vi "Set Remote Sensors.vi"(10 "Robot Sensors In":T1[](array[typedef]) {"Kobuki Sensors"."Infrared" format="%02x"; "iRobot Sensors"."Infrared" format="%02x"; "accelerometer"."z axis (g)" format="%.3f"; "accelerometer"."y axis (g)" format="%.3f"; "accelerometer"."x axis (g)" format="%.3f"}, 11 "Communication Refs":T14[](array[typedef])) -> ()   [LabVIEW 2014]
uses:
  iRobot Remote Ref.ctl
  iRobot/Sensor/Sensor Group 6.ctl
  iRobot/Sensor/Bumps + Wheel Drops.ctl
  iRobot/Sensor/Buttons.ctl
  iRobot/Sensor/Charging State.ctl
  iRobot/Sensor/Charging Sources Available.ctl
  iRobot/Sensor/OI Mode.ctl
  iRobot/Sensor/Cargo Bay Digital Inputs.ctl
  iRobot/Sensor/Low-Side Driver + Wheel Overcurrent.ctl
  shared/Sensors.ctl
  iRobot/Sensor/Accelerometer.ctl
  Kobuki/KobukiSensors.ctl
  Kobuki/Kobuki Bumps and WheelDrops.ctl
  Kobuki/Kobuki Buttons.ctl
panel:
  # "Electrical: charging, battery, OI mode"
  # "Sensors: bump, cliff, button, wheel drop, wall, virtual wall"
  # "Motion: distance, angle, requested velocity"
  # "Cargo Bay: I/O, overcurrent, infrared"
  # "Song"
  # "Electrical: charging, battery, OI mode"
  # "Sensors: bump, cliff, button, wheel drop, wall, virtual wall"
  # "Motion: distance, angle, requested velocity"
  # "Cargo Bay: I/O, overcurrent, infrared"
  # "Song"
  # "Electrical: charging, battery, OI mode"
  # "Sensors: bump, cliff, button, wheel drop, wall, virtual wall"
  # "Motion: distance, angle, requested velocity"
  # "Cargo Bay: I/O, overcurrent, infrared"
  # "Song"
  # "Electrical: charging, battery, OI mode"
  # "Sensors: bump, cliff, button, wheel drop, wall, virtual wall"
  # "Motion: distance, angle, requested velocity"
  # "Cargo Bay: I/O, overcurrent, infrared"
  # "Song"
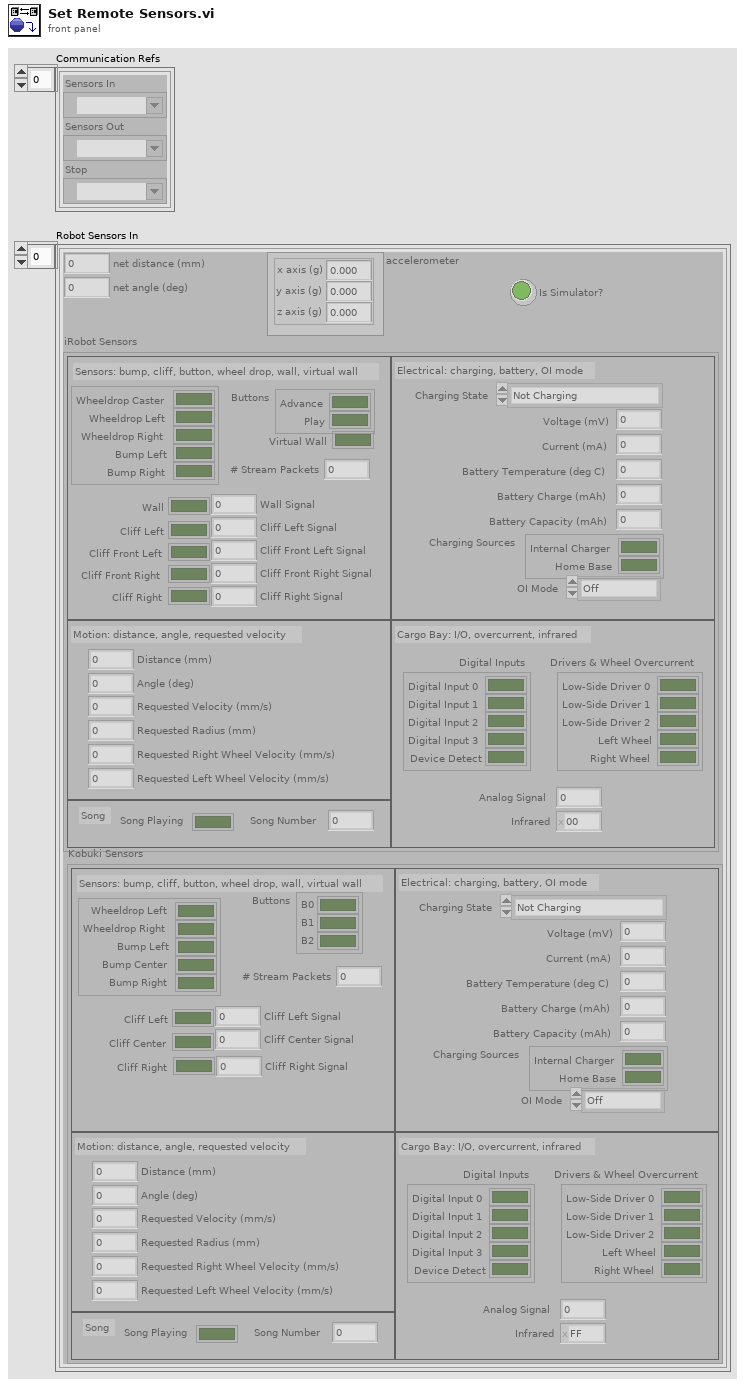
[diagram p1: front panel]
types:
  T1 = typedef "Sensors.ctl" = cluster{"net distance (mm)":i32, "net angle (deg)":i32, "accelerometer":T2, "iRobot Sensors":T3, "Is Simulator?":bool, "Kobuki Sensors":T11}
  T2 = typedef "Accelerometer.ctl" = cluster{"x axis (g)":dbl, "y axis (g)":dbl, "z axis (g)":dbl}
  T3 = typedef "Sensor Group 6.ctl" = cluster{"Bumps + Wheel Drops":T4, "Wall":bool, "Cliff Left":bool, "Cliff Front Left":bool, "Cliff Front Right":bool, "Cliff Right":bool, "Wall Signal":u16, "Cliff Left Signal":u16, "Cliff Front Left Signal":u16, "Cliff Front Right Signal":u16, "Cliff Right Signal":u16, "Buttons":T5, "Virtual Wall":bool, "# Stream Packets":u8, "Requested Velocity (mm/s)":i16, "Requested Radius (mm)":i16, "Requested Right Wheel Velocity (mm/s)":i16, "Requested Left Wheel Velocity (mm/s)":i16, "Distance (mm)":i32, "Angle (deg)":i32, "Song Playing":bool, "Song Number":u8, "Charging State":T6, "Voltage (mV)":u16, "Current (mA)":i16, "Battery Temperature (deg C)":i8, "Battery Charge (mAh)":u16, "Battery Capacity (mAh)":u16, "Charging Sources":T7, "OI Mode":T8, "Digital Inputs":T9, "Drivers & Wheel Overcurrent":T10, "Analog Signal":u16, "Infrared":u8}
  T4 = typedef "Bumps + Wheel Drops.ctl" = cluster{"Wheeldrop Caster":bool, "Wheeldrop Left":bool, "Wheeldrop Right":bool, "Bump Left":bool, "Bump Right":bool}
  T5 = typedef "Buttons.ctl" = cluster{"Advance":bool, "Play":bool}
  T6 = typedef "Charging State.ctl" = enum16{"Not Charging", "Reconditioning Charging", "Full Charging", "Trickle Charging", "Waiting", "Charging Fault Condition"}
  T7 = typedef "Charging Sources Available.ctl" = cluster{"Internal Charger":bool, "Home Base":bool}
  T8 = typedef "OI Mode.ctl" = enum16{"Off", "Passive", "Safe", "Full"}
  T9 = typedef "Cargo Bay Digital Inputs.ctl" = cluster{"Digital Input 0":bool, "Digital Input 1":bool, "Digital Input 2":bool, "Digital Input 3":bool, "Device Detect":bool}
  T10 = typedef "Low-Side Driver + Wheel Overcurrent.ctl" = cluster{"Low-Side Driver 0":bool, "Low-Side Driver 1":bool, "Low-Side Driver 2":bool, "Left Wheel":bool, "Right Wheel":bool}
  T11 = typedef "KobukiSensors.ctl" = cluster{"Bumps + Wheel Drops":T12, "Cliff Left":bool, "Cliff Center":bool, "Cliff Right":bool, "Cliff Left Signal":u16, "Cliff Center Signal":u16, "Cliff Right Signal":u16, "Buttons":T13, "# Stream Packets":u8, "Requested Velocity (mm/s)":i16, "Requested Radius (mm)":i16, "Requested Right Wheel Velocity (mm/s)":i16, "Requested Left Wheel Velocity (mm/s)":i16, "Distance (mm)":i32, "Angle (deg)":i32, "Song Playing":bool, "Song Number":u8, "Charging State":T6, "Voltage (mV)":u16, "Current (mA)":i16, "Battery Temperature (deg C)":i8, "Battery Charge (mAh)":u16, "Battery Capacity (mAh)":u16, "Charging Sources":T7, "OI Mode":T8, "Digital Inputs":T9, "Drivers & Wheel Overcurrent":T10, "Analog Signal":u16, "Infrared":u8}
  T12 = typedef "Kobuki Bumps and WheelDrops.ctl" = cluster{"Wheeldrop Left":bool, "Wheeldrop Right":bool, "Bump Left":bool, "Bump Center":bool, "Bump Right":bool}
  T13 = typedef "Kobuki Buttons.ctl" = cluster{"B0":bool, "B1":bool, "B2":bool}
  T14 = typedef "iRobot Remote Ref.ctl" = cluster{"Sensors In":refnum<k21>, "Sensors Out":refnum<k21>, "Stop":refnum<k21>}
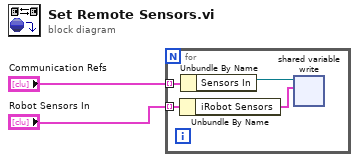
[diagram p0: block diagram]
diagram:
  n1 = for {
    tunnel: "Robot Sensors In" -> [w4] mode=indexing
    tunnel: "Communication Refs" -> [w6] mode=indexing
    n2 = Unbundle By Name(w4) -> ("iRobot Sensors"=w3:T3)
    n3 = Unbundle By Name(w6) -> ("Sensors In"=w5:refnum<k21>)
    n4 = shared-variable-write(w5, w3) -> ()  [unwired: 1 in, 2 out]
  }
